vi "Read settings.vi"(8 "error in (no error)":errorcluster, 9 "force loading?":bool=TRUE, 10 "settings name":string, 11 "ImagingModeSPIM in":refnum<class "InVivo_ImagingModeSPIM.lvclass">) -> (0 "error out":errorcluster, 1 "loaded?":bool, 2 "setting name":string, 3 "ImagingModeSPIM out":refnum<class "InVivo_ImagingModeSPIM.lvclass">)   [LabVIEW 2012, in "InVivo_ImagingModeSPIM.lvclass"]
uses:
  InVivo_ImagingModeSPIM.lvclass
  <vilib>/Distrio/Murmex/Murmex/Murmex.lvclass
  InVivo_ImagingModeSPIM.lvclass/InVivo_ImagingModeSPIM.ctl
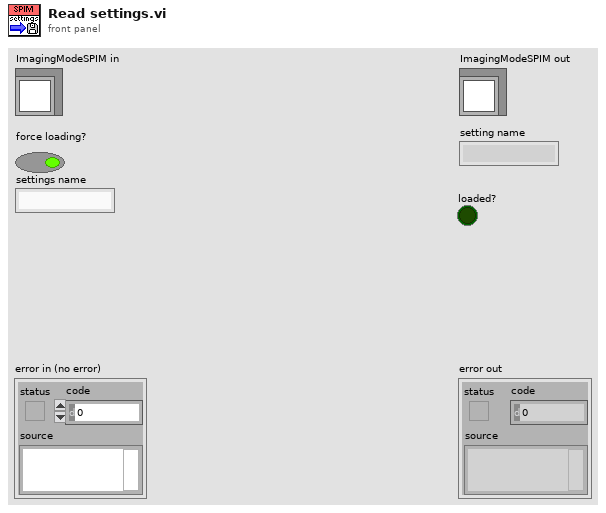
[diagram p1: front panel]
types:
  T1 = typedef "InVivo_ImagingModeSPIM.lvclass/settings_cluster.ctl" = cluster{"Frequency":dbl[unit], "Amplitude1":dbl[unit], "Phase1":dbl[unit], "DC offset1":dbl[unit], "Amplitude2":dbl[unit], "Phase2":dbl[unit], "DC offset2":dbl[unit], "Waveform type":T2, "HSYNC pulses":i32, "pulses per pixel":i32, "digital ratio":dbl, "DC offset3":dbl[unit], "Amplitude3":dbl[unit], "Phase3":dbl[unit], "AOTFamplitude":dbl[unit], "AOTFoffset":dbl[unit], "AOTFphase":dbl[unit]}
  T2 = typedef "InVivo_ImagingModeSPIM.lvclass/waveform_enum.ctl" = enum16{"triangular", "sawtooth", "sinusodial"}
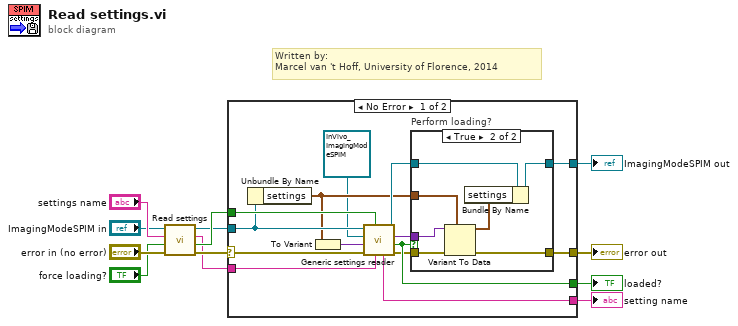
[diagram p0: block diagram]
diagram:
  # "Written by:\nMarcel van 't Hoff, University of Florence, 2014"
  n1 = call-parent "Read settings.vi"("error in (no error)"="error in (no error)", "force loading?"="force loading?", "settings name"="settings name", "Murmex in"="ImagingModeSPIM in") -> ("error out"=w8:errorcluster, "loaded?"=w7:bool, "setting name"=w6:string, "Murmex out"=w5:refnum<class "InVivo_ImagingModeSPIM.lvclass">)  [unwired: 4 in]
  n2 = case shown="No Error" w8 {
    selector: w8 -> [w23 w37]
    tunnel: [w25 w37] -> w4
    tunnel: [w26 w36] -> w3
    tunnel: w5 -> [w22 w36]
    tunnel: w7 -> [w24 _]
    tunnel: [w21 _] -> w1
    tunnel: w6 -> [w20 _]
    tunnel: [w19 _] -> w2
    frame No Error {
      n3 = Unbundle By Name(w22) -> ("settings"=w15:T1)
      n4 = To Variant(anything=w15) -> (Variant=w16:variant)
      n5 = call <vilib>:"Generic settings reader.vi"("settings name"=w20, "force loading?"=w24, "error in (no error)"=w23, "settings cluster variant"=w16, "inheritance level"=refnum<class "InVivo_ImagingModeSPIM.lvclass"> refnum ("ImagingModeSPIM"), "Murmex in"=w22) -> ("error out"=w18:errorcluster, "loaded?"=w19:bool, "settings data (variant)"=w14:variant, "Murmex out"=w17:refnum<class "InVivo_ImagingModeSPIM.lvclass">, "setting name"=w21:string)  [unwired: 1 in]
      n6 = case "Perform loading?" shown="True" w19 {
        tunnel: [w28 w29] -> w26
        tunnel: w15 -> [_ w35]
        tunnel: [w27 w30] -> w25
        tunnel: w18 -> [w27 w32]
        tunnel: w17 -> [w28 w34]
        tunnel: w14 -> [_ w31]
        frame False {
        }
        frame True {
          n7 = Variant To Data(error in=w32, type=w35, Variant=w31) -> (data=w33:T1, error out=w30:errorcluster)
          n8 = Bundle By Name(cluster=w34, "settings"=w33) -> (w29:refnum<class "InVivo_ImagingModeSPIM.lvclass">)
        }
      }
    }
    frame Error {
    }
  }
  "error out" <- w4
  "ImagingModeSPIM out" <- w3
  "setting name" <- w1
  "loaded?" <- w2
